vi "Request.vi"(8 "error in (no error)":errorcluster, 11 "Controller Data Cluster":T1={"UI Data Cluster"={"Floor Selection"=[], "Elevator Call Up"=[], "Elevator Call Down"=[], "Door Buttons"={"Open"=FALSE, "Close"=FALSE}, "Emergency"=FALSE}, "Sensor Position"=1, "Module Closed?"={"Display Loop"=FALSE, "Sensor Loop "=FALSE}, "Time to Elapse"=0, "Request?"=FALSE, "Timed Action"=enum."Open Door", "Time Constants"={"Open Door"=5.0, "Close Door"=1.0, "Travel"=10.0, "Inactivity"=20.0}, "Inactivity"=FALSE, "Current Floor"=1, "Current Direction"=enum."Idle", "Travel?"=FALSE, "Program Exit"=[], "Emergency?"=FALSE}) -> (0 "error out":errorcluster, 3 "Request?":bool)   [LabVIEW 2017]
uses:
  Controller Data Cluster.ctl
  User Console/UI Data Cluster.ctl
  Timed Action.ctl
  Current Direction.ctl
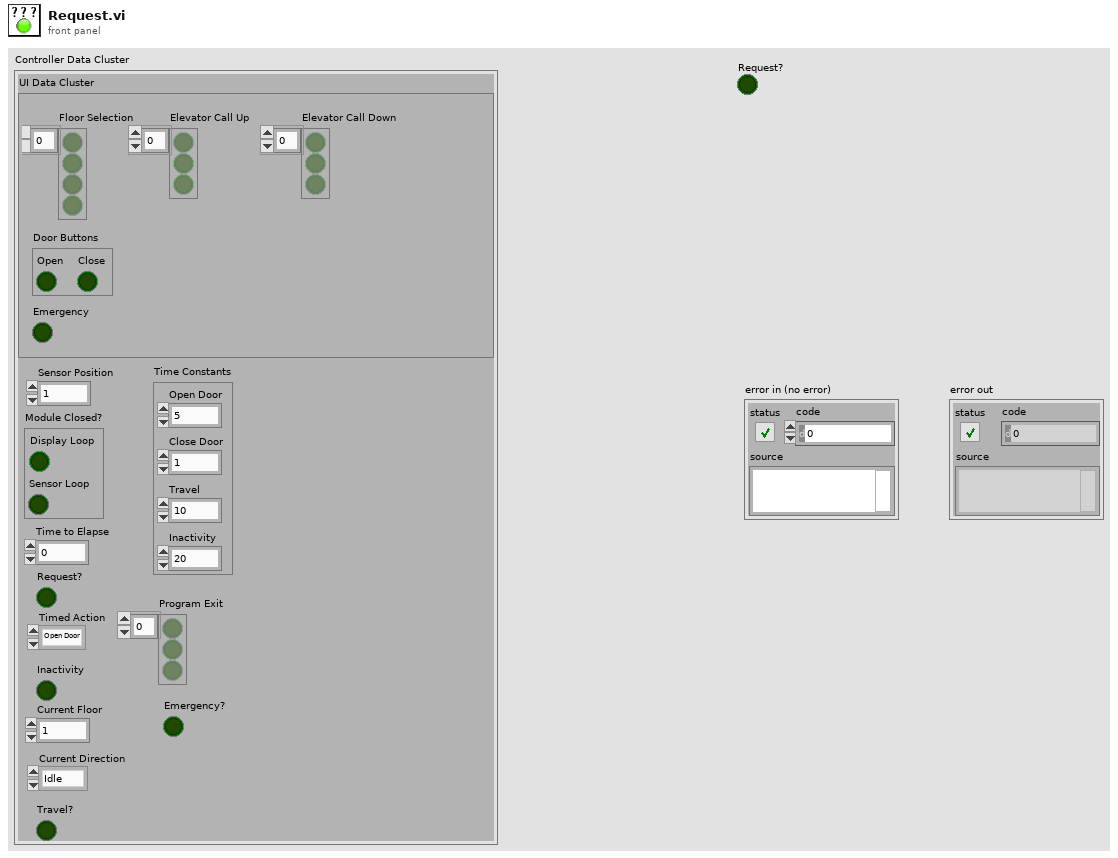
[diagram p1: front panel]
types:
  T1 = typedef "Controller Data Cluster.ctl" = cluster{"UI Data Cluster":T2, "Sensor Position":u32, "Module Closed?":cluster{"Display Loop":bool, "Sensor Loop ":bool}, "Time to Elapse":u32, "Request?":bool, "Timed Action":T3, "Time Constants":cluster{"Open Door":dbl, "Close Door":dbl, "Travel":dbl, "Inactivity":dbl}, "Inactivity":bool, "Current Floor":u32, "Current Direction":T4, "Travel?":bool, "Program Exit":bool[], "Emergency?":bool}
  T2 = typedef "UI Data Cluster.ctl" = cluster{"Floor Selection":bool[], "Elevator Call Up":bool[], "Elevator Call Down":bool[], "Door Buttons":cluster{"Open":bool, "Close":bool}, "Emergency":bool}
  T3 = typedef "Timed Action.ctl" = enum16{"Open Door", "Close Door", "Travel", "Inactivity"}
  T4 = typedef "Current Direction.ctl" = enum16{"Up", "Down", "Idle"}
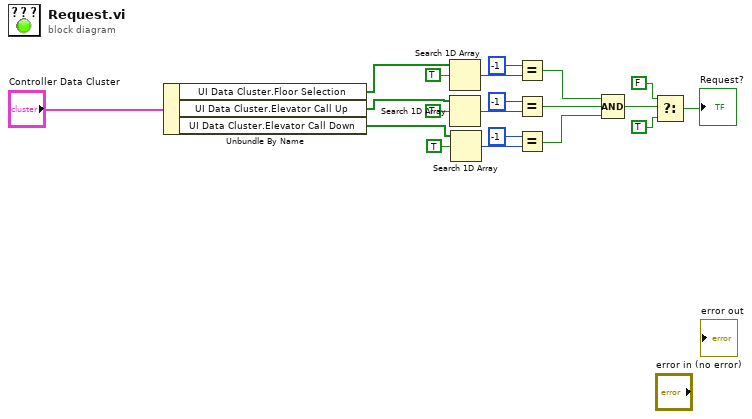
[diagram p0: block diagram]
diagram:
  n1 = Unbundle By Name("Controller Data Cluster") -> ("UI Data Cluster.Floor Selection"=w19:bool[], "UI Data Cluster.Elevator Call Up"=w15:bool[], "UI Data Cluster.Elevator Call Down"=w14:bool[])
  n2 = Search 1D Array(1D array=w19, element=TRUE) -> (index of element=w13:i32)  [unwired: 1 in]
  n3 = Search 1D Array(1D array=w15, element=TRUE) -> (index of element=w10:i32)  [unwired: 1 in]
  n4 = Search 1D Array(1D array=w14, element=TRUE) -> (index of element=w8:i32)  [unwired: 1 in]
  n5 = Equal?(x=-1, y=w13) -> (x = y?=w7:bool)
  n6 = Equal?(x=-1, y=w10) -> (x = y?=w6:bool)
  n7 = Equal?(x=-1, y=w8) -> (x = y?=w5:bool)
  n8 = Compound Arithmetic op=AND(w7, w6, w5) -> (w4:bool)
  n9 = Select(t=FALSE ("element"), s=w4, f=TRUE ("element")) -> (s? t:f=→"Request?":bool)
